vi "ECS-Diesel-Host.vi"() -> ()   [LabVIEW 2015]
uses:
  <vilib>/addons/Software Calibration Management/XControls/SubHost.xctl
  <vilib>/addons/Software Calibration Management/XControls/SubHost List.xctl
  Typedefs/EPT/Engine Status.ctl
  SubHosts/Support/Tracking Chart xCTL/TrackingChart.xctl
  <vilib>/addons/Software Calibration Management/XControls/TBL1D.xctl
  <vilib>/addons/Software Calibration Management/XControls/Faults.xctl
  ECS-Host.lvlib
  ECS-Shared.lvlib
panel:
  out "CalPointData":sgl[](array[numeric])
  in  "_Refresh":bool
  in  "EngineSpeed_MaxNC":sgl
  in  "EngineSpeed_MaxCrit":sgl
  out "5VPSU_CriticalFault":bool
  out "12VPSU_CriticalFault":bool
  out "BattV_CriticalFault":bool
  in  "_Main Tabs":T1(tab)
  in  "PowerEnable":bool caption="Power Enable"
  out "EngineSpeedFPGA1":sgl(knob) scale=0.0..1000.0 scale format="%#_6p"
  in  "SyncEnable":bool caption="Sync Enable"
  out "ReceivingPrimaryFPGA1":bool caption="Rcvg Primary"
  out "SyncFPGA1":bool caption="Sync"
  out "_BattVPresent":bool caption="Battery"
  out "_12VPresent":bool caption="12V"
  out "_5VPresent":bool caption="5V"
  out "Engine Time":sgl caption="[hr]" format="%0#5_4f"
  out "Time Since Start":sgl caption="[sec]" format="%05.0f"
  in  "Engine Time Reset":bool
  out "_Engine Speed":sgl format="%#.0f"
  out "Software Version":string caption="Version:"
  out "_Engine Status":T2 caption="Engine Status"
  in  "Faults Table":T4(xcontrol)
  in  "_SubHost Tab":T5(tab)
  in  "XNET CAN":T6(xcontrol)
  in  "Power":T6(xcontrol)
  in  "TDK High Voltage Supply":T6(xcontrol)
  in  "NI 9754-1 (ESTTL)":T6(xcontrol)
  in  "NI 9411-1 (Digital Input)":T6(xcontrol)
  in  "NI 9758-2 (PFI/LS)":T6(xcontrol)
  in  "NI 9751-4 (DI Driver)":T6(xcontrol)
  in  "NI 9751-3 (DI Driver)":T6(xcontrol)
  in  "NI 9751-2 (DI Driver)":T6(xcontrol)
  in  "NI 9752-1 (ADCombo)":T6(xcontrol)
  in  "NI 9757-1 (O2)":T6(xcontrol)
  in  "NI 9755-1 (NOx)":T6(xcontrol)
  in  "NI 9759-1 (Throttle)":T6(xcontrol)
  in  "NI 9758-1 (PFI/LS)":T6(xcontrol)
  in  "NI 9751-1 (DI Driver)":T6(xcontrol)
  in  "EPTx":T6(xcontrol)
  in  "Sensors":T6(xcontrol)
  in  "Faults":T6(xcontrol) caption="0"
  in  "Engine Specs":T6(xcontrol)
  in  "High Pressure Common Rail":T6(xcontrol)
  in  "Variable Valve Actuation":T6(xcontrol)
  in  "Boost Actuation":T6(xcontrol)
  in  "Direct Injectors":T6(xcontrol)
  in  "EGR Actuation":T6(xcontrol)
  in  "EGR Control":T6(xcontrol) caption="5"
  in  "Cranking":T6(xcontrol) caption="0"
  in  "Wastegate Control":T6(xcontrol) caption="6"
  in  "VGT Control":T6(xcontrol) caption="6"
  in  "Intake Air Desired MAP":T6(xcontrol) caption="5"
  in  "DI Control":T6(xcontrol) caption="2"
  in  "Fuel Command":T6(xcontrol) caption="1"
  in  "Load Command":T6(xcontrol) caption="0"
  in  "Intake Air Measured":T6(xcontrol) caption="1"
  in  "EGR Flow":T6(xcontrol) caption="5"
  in  "VVT/VVA Control":T6(xcontrol) caption="9"
  in  "Rail Pressure Control":T6(xcontrol) caption="4"
  in  "Execution Info":T6(xcontrol)
  in  "Calscope and Trends":T6(xcontrol)
  in  "_HiddenControls":enum32{"Page 1"}(tab)
  out "RailP_Des":sgl
  out "MAP_Des":sgl
  in  "NominalMEP_Tbl":cluster{"X":sgl[], "Y":sgl[]}(xcontrol)
  out "MEP_Des":sgl caption="EngineLoad_Des"
  out "Pedal_Des":sgl
  out "EngineStatus":u8
  in  "_HiddenControls2":enum32{"Page 1"}(tab)
  in  "SliderMin":sgl[](array[numeric])
  in  "SliderMax":sgl[](array[numeric])
  in  "Units":string
  in  "_Signal Names":string[](array[string])
  in  "CalPointIDs":sgl[](array[numeric])
  out "NamesLong":string
  in  "SliderSelection":sgl[](array[numeric])
  in  "MAP_ManE":bool
  in  "Pedal_ManE":bool
  in  "MEP_ManE":bool
  in  "RailP_ManE":bool
  in  "Pedal_Man":sgl(slide) caption="[bar]" scale=0.0..100.0 scale format="%#4.1f"
  in  "MEP_Man":sgl(slide) caption="[bar]" scale=0.0..25.0 scale format="%#4.1f"
  in  "RailP_Man":sgl(slide) caption="[bar]" scale=0.0..2000.0 scale format="%#4.1f"
  in  "MAP_Man":sgl(slide) caption="[kPa]" scale=0.0..400.0 scale format="%#4.1f"
  in  "ForceSafeState":bool caption="Push to Force Safe State"
  out "Non-Critical Fault":bool
  out "Critical Fault":bool
  in  "ESTOP":bool caption="Push to Stop"
  in  "System":T7(xcontrol)
  in  "Control":T7(xcontrol)
  in  "Engine":T7(xcontrol)
  in  "Hardware":T7(xcontrol)
  out "_TrackingChart":T8(xcontrol)
  in  "_Delete":bool
  in  "_Down":bool
  in  "_Up":bool
  in  "_Insert":bool
  out "_Data (Hidden)":string[](array[string])
  in  "_Units":string caption="Units"
  in  "_Slider Max":sgl caption="Max"
  in  "_Slider Min":sgl caption="Min"
  in  "_CalpointIDSelect":u16(ring) caption="Signal Name"
  in  "_Slider Selection":T9(ring) caption="Slider Selection"
  in  "_Table":i32(listbox)
  in  "_Chart History1":i32=20 caption="Chart History"
  out "_LoadTracking":cluster{"X Buffer":sgl[], "Y Buffer":sgl[]}[](graph) caption="Load Tracking"
  in  "_Chart History2":i32=20 caption="Chart History"
  in  "_Normalize":bool=TRUE caption="Normalize"
  in  "_Var Select":u16(ring) caption="Signal Selection" items=["EngineLoad_Des", "InjDur", "InjTiming", "RailP", "RailP_Des", "MAP", "MAP_Des", "MAF", "Lambda", "FuelT", "ECT", "MAT", "OilP", "ExhaustManifoldT", "MainSpkDwell", "MainSpkTiming"]
  out "_ReturnMap":cluster{"X Buffer":sgl[], "Y Buffer":sgl[]}[](graph) caption="Return Map"
  # "Engine Control System"
  # "RPM"
  # "Customize UI Here"
  # "Customize UI Here"
  # "Customize UI Here"
  # "Un-hide from the block diagram by right-clicking '_HiddenControls' and selecting 'Show Control'"
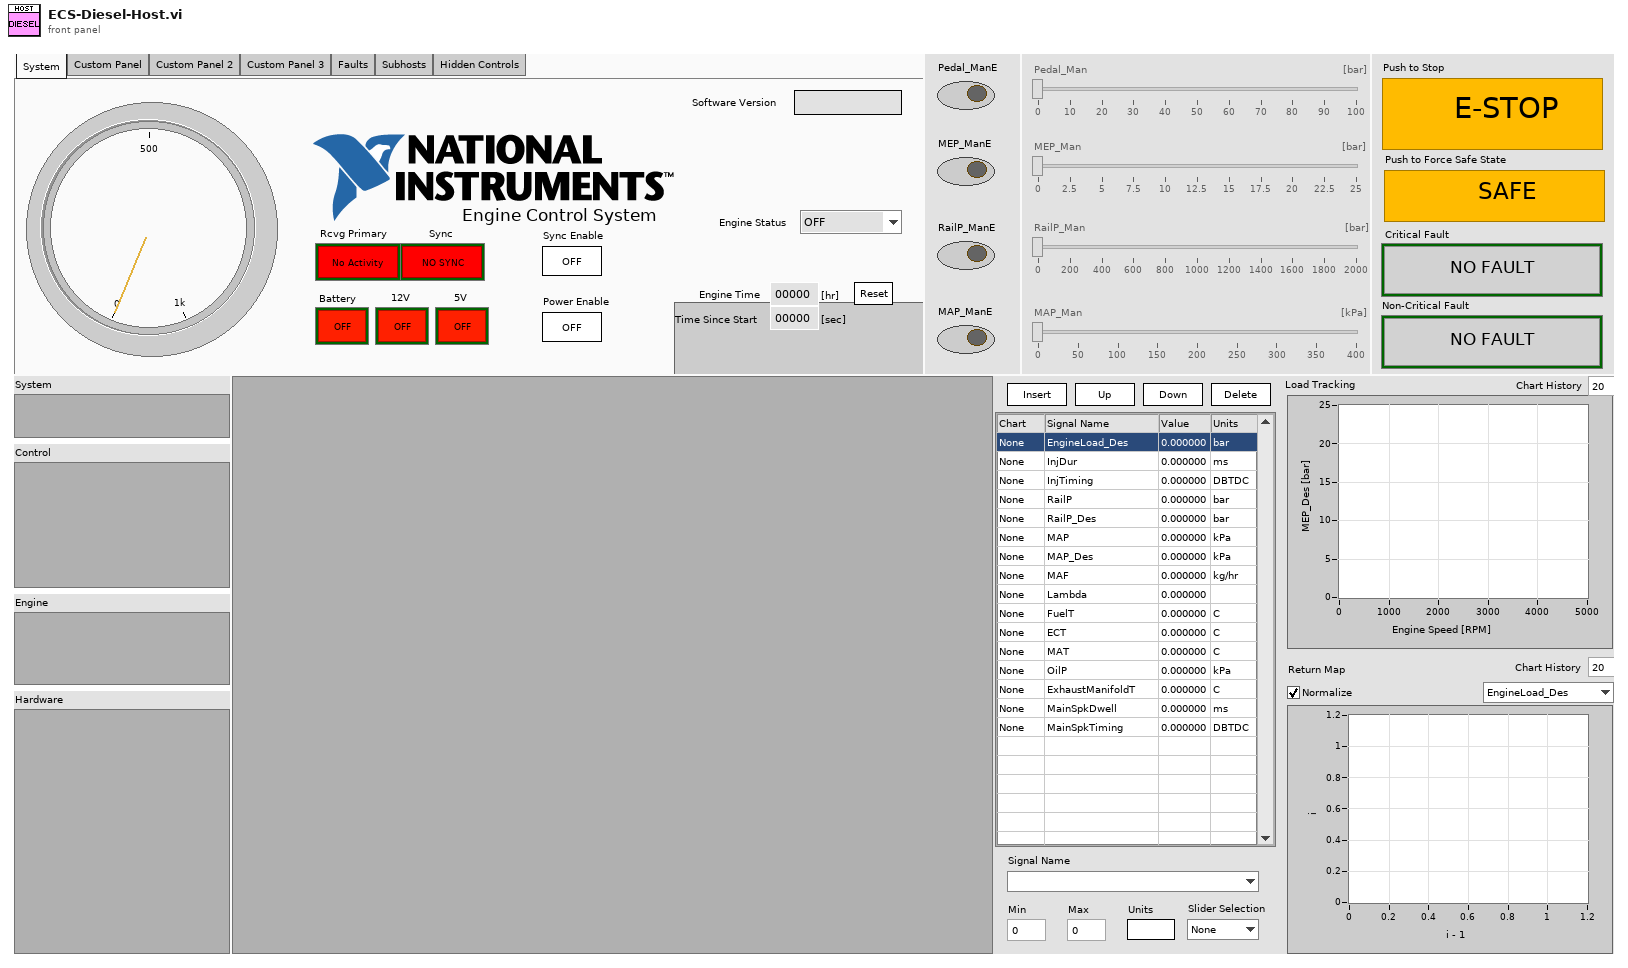
[diagram p1: front panel]
types:
  T1 = enum32{"System", "Custom Panel", "Custom Panel 2", "Custom Panel 3", "Faults", "Subhosts", "Hidden Controls"}
  T2 = typedef "ECS-Shared.lvlib/Engine Status.ctl" = enum16{"OFF", "STALLED", "CRANKING", "RUNNING", "ACCEL", "DECEL", "SAFE"}
  T3 = typedef "Faults.xctl/Faults - Active.ctl" = cluster{"Highest Level":i32, "Very Low":u32, "Low":u32, "Medium":u32, "High":u32, "Very High":u32}
  T4 = cluster{"Active Faults":T3, "Unacknowledged Faults":T3}
  T5 = enum32{"Hardware I/O", "Engine I/O", "Control", "System"}
  T6 = cluster{"Name":string, "Host VI":path, "Pairing File":path, "Display Name":string}
  T7 = cluster{"States":enum32{"Invalid", "Standard", "Closed", "Hidden", "Minimized", "Maximized"}[], "VI Names":string[], "VI Refnums":refnum<vi>[], "Sub-Host Group":string, "Scrollbar":bool, "Listbox":refnum<vi>}
  T8 = cluster{"Value":sgl, "Name":string, "Unit":string, "Max":sgl, "Min":sgl}[]
  T9 = enum16{"None", "Slider 1", "Slider 2", "Slider 3", "Slider 4"}
  T10 = enum8{"Enabled", "Disabled", "Disabled and Grayed Out"}
  T11 = cluster{"Value":sgl, "Name":string, "Unit":string, "Max":sgl, "Min":sgl}
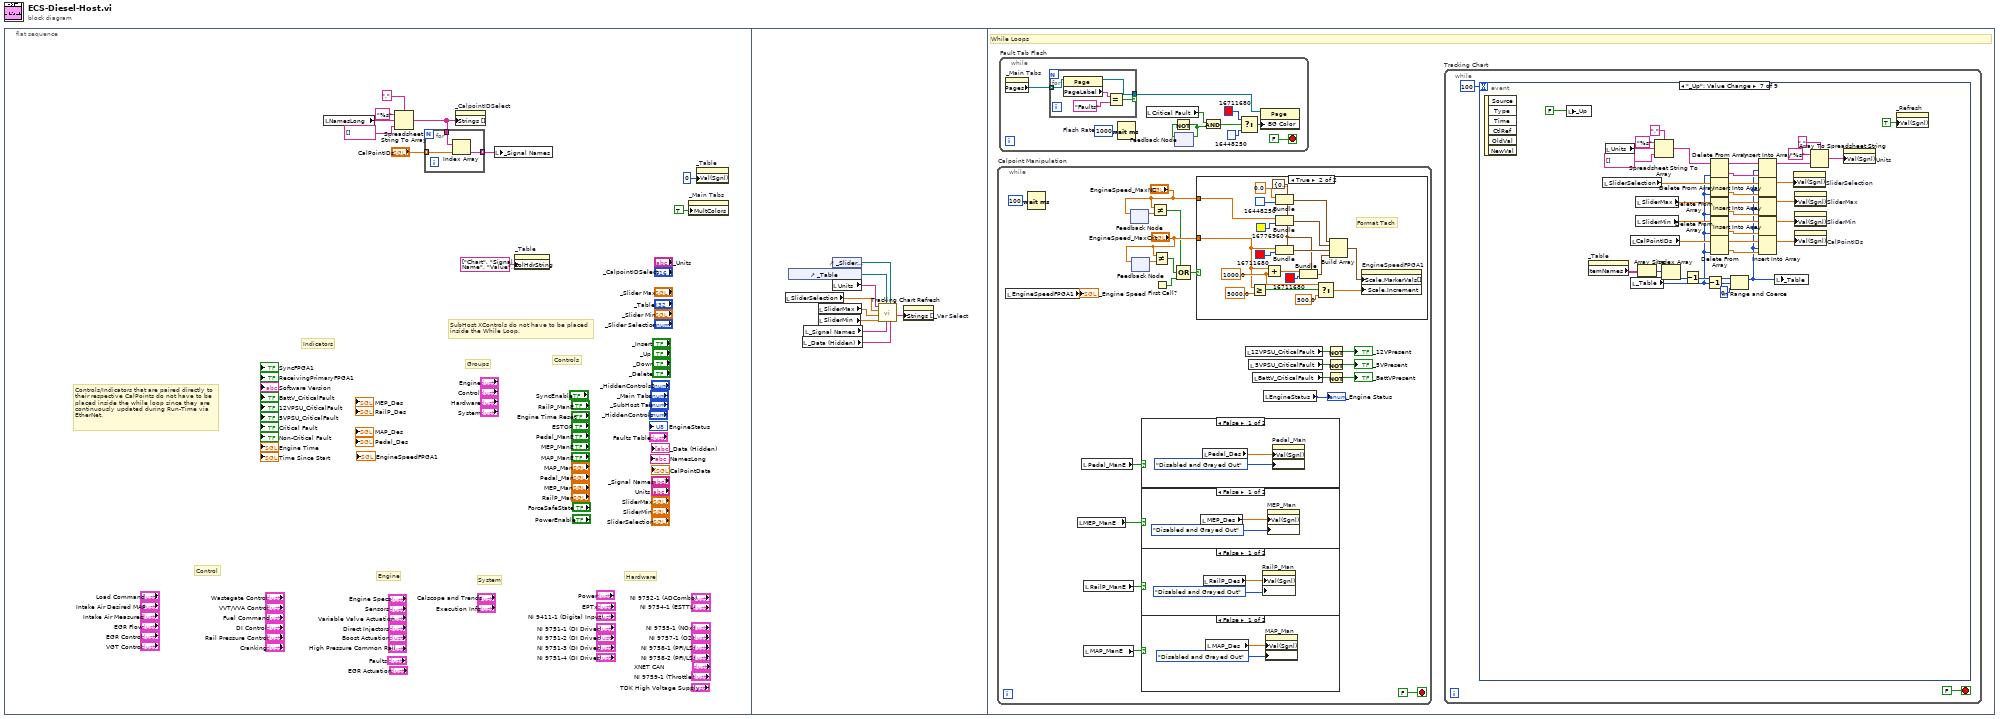
[diagram p0: block diagram]
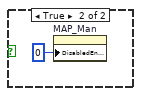
[diagram p2: hidden frame]
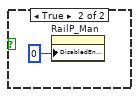
[diagram p3: hidden frame]
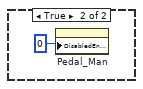
[diagram p4: hidden frame]
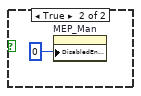
[diagram p5: hidden frame]
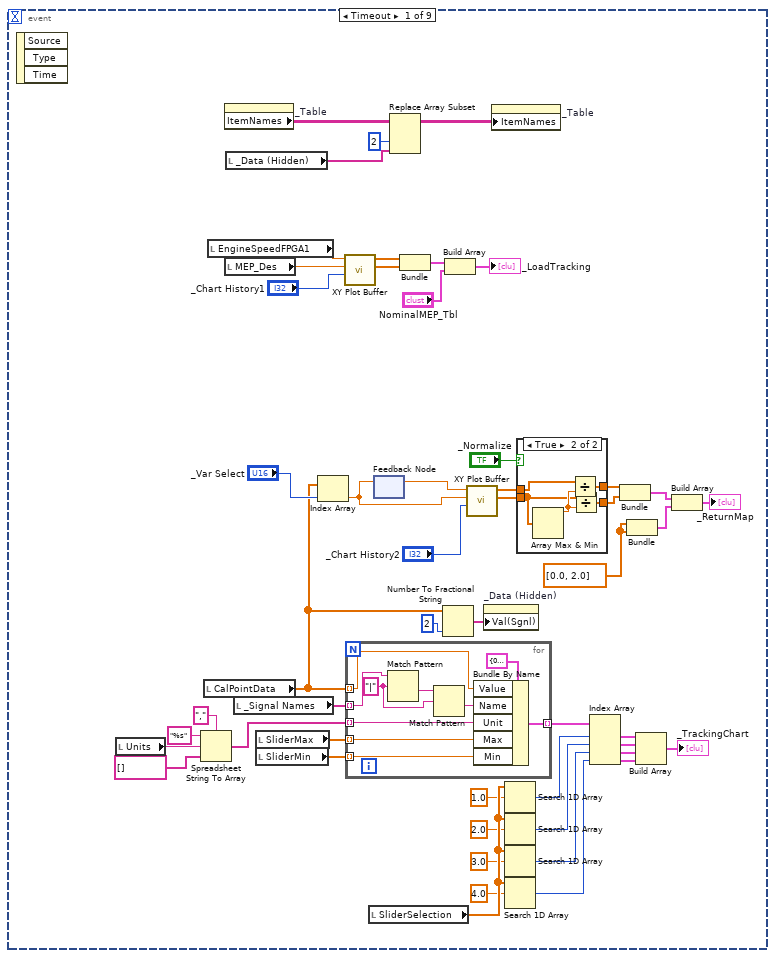
[diagram p7: hidden frame]
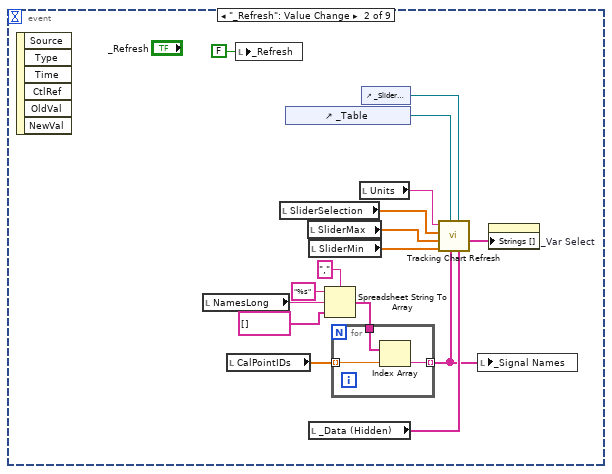
[diagram p9: hidden frame]
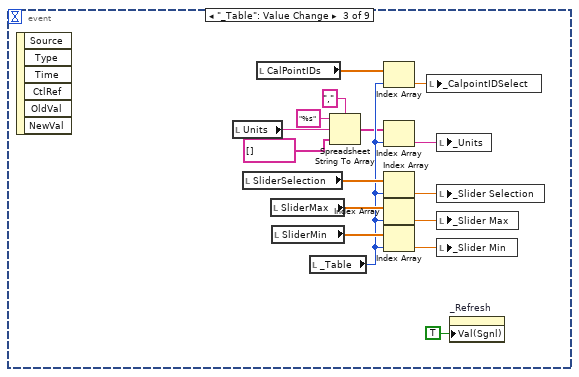
[diagram p10: hidden frame]
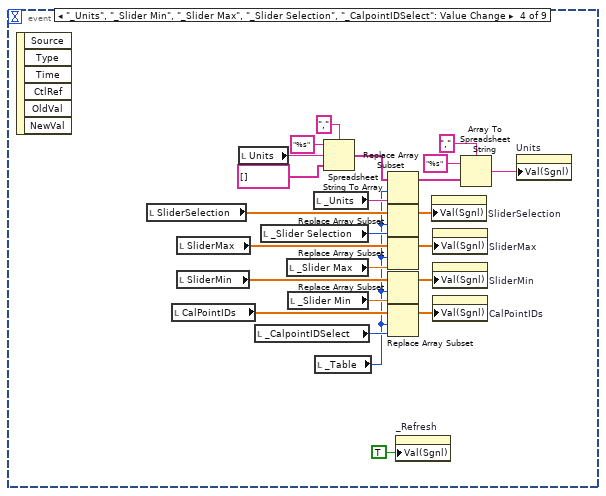
[diagram p11: hidden frame]
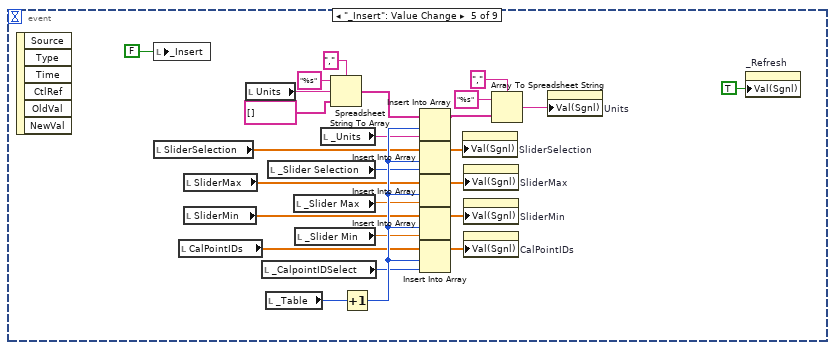
[diagram p12: hidden frame]
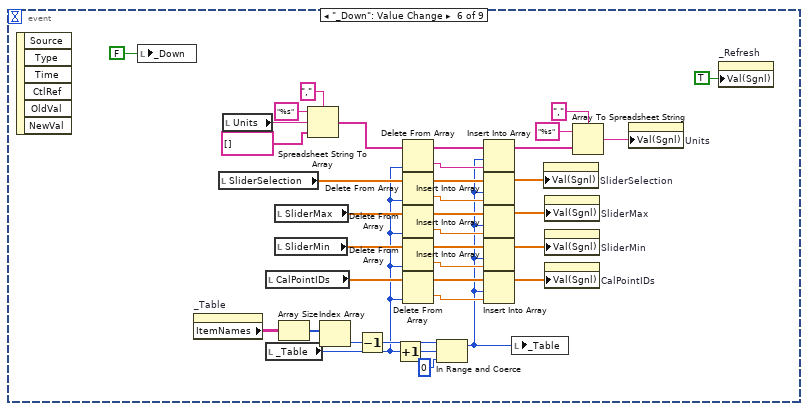
[diagram p13: hidden frame]
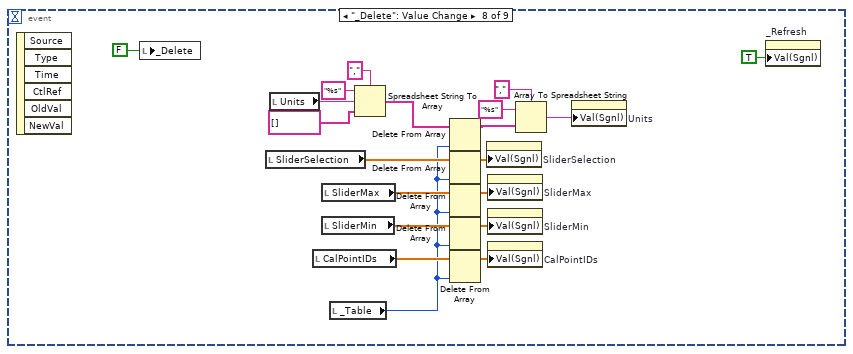
[diagram p14: hidden frame]
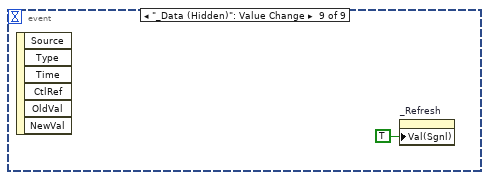
[diagram p15: hidden frame]
diagram:
  n1 = flat-sequence {
    frame #0 {
      # "System"
      # "Hardware"
      # "Engine"
      # "Control"
      # "Controls"
      # "Indicators"
      # "Groups"
      # "Controls/Indicators that are paired directly to their respective CalPoints do not have to be placed inside the while loop since they are continuously updated during Run-Time via EtherNet."
      # "SubHost XControls do not have to be placed inside the While Loop."
      n2 = local read "NamesLong"() -> (w4:string)
      n3 = Spreadsheet String To Array(delimiter (Tab)=",", format string="%s", spreadsheet string=w4, array type (2D Dbl)=string[] []) -> (array=w1:string[])
      n4 = for {
        tunnel: "CalPointIDs" -> [w13] mode=indexing
        tunnel: w1 -> [w12]
        tunnel: [w11] -> w2 mode=indexing
        n5 = Index Array(array=w12, index=w13) -> (element=w11:string)
      }
      n6 = property on="_CalpointIDSelect" class="Ring (strict)"("Strings []"=w1) -> ()  [unwired: 2 in, 2 out]
      n7 = local write "_Signal Names"(w2) -> ()
      n8 = property on="_Table" class="MCListbox (strict)"("ColHdrString"=string[] ["Chart", "Signal Name", "Value", "Units"] ("Column Header Strings[]")) -> ()  [unwired: 2 in, 2 out]
      n9 = property on="_Main Tabs" class="TabCtl (strict)"("MultColors"=TRUE ("Allow Multiple Colors")) -> ()  [unwired: 2 in, 2 out]
      n10 = property on="_Table" class="MCListbox (strict)"("Val(Sgnl)"=0 ("Value (Signaling)")) -> ()  [unwired: 2 in, 2 out]
    }
    frame #1 {
      n11 = local read "SliderSelection"() -> (w20:sgl[])
      n12 = control-ref of="_Table"() -> (w21:refnum<vi>)
      n13 = local read "_Data (Hidden)"() -> (w17:string[])
      n14 = local read "_Signal Names"() -> (w16:string[])
      n15 = local read "SliderMax"() -> (w19:sgl[])
      n16 = local read "SliderMin"() -> (w18:sgl[])
      n17 = local read "Units"() -> (w15:string)
      n18 = control-ref of="_Slider Selection"() -> (w22:refnum<vi>)
      n19 = call "Tracking Chart Refresh.vi"("Data"=w17, "_Slider Selection"=w22, "Signal Names"=w16, "_Table"=w21, "Slider Min"=w18, "Slider Max"=w19, "Slider Selections"=w20, "Units"=w15) -> ("Short Signal Names"=w14:string[])  [unwired: 3 in]
      n20 = property on="_Var Select" class="Ring (strict)"("Strings []"=w14) -> ()  [unwired: 2 in, 2 out]
    }
    frame #2 {
      # "While Loops"
      n21 = while "Calpoint Manipulation" {
        stop <- FALSE stop-if-true
        n22 = local read "EngineSpeedFPGA1"() -> (→"_Engine Speed":sgl)
        n23 = Wait (ms)(milliseconds to wait=u32 100) -> ()  [unwired: 1 out]
        n24 = local read "MEP_ManE"() -> (w43:bool)
        n25 = local read "Pedal_ManE"() -> (w42:bool)
        n26 = local read "RailP_ManE"() -> (w41:bool)
        n27 = local read "MAP_ManE"() -> (w40:bool)
        n28 = feedback #1() -> (w49:sgl)  [unwired: 1 in]
        n29 = feedback-in #1("EngineSpeed_MaxNC") -> ()
        n30 = feedback #2() -> (w57:sgl)  [unwired: 1 in]
        n31 = feedback-in #2("EngineSpeed_MaxCrit") -> ()
        n32 = case shown="False" w42 {
          frame False {
            n33 = local read "Pedal_Des"() -> (w67:sgl)
            n34 = property on="Pedal_Man" class="Slide (strict)"("Val(Sgnl)"=w67, "DisabledEnum"=T10."Disabled and Grayed Out" ("Disabled")) -> ()  [unwired: 2 in, 2 out]
          }
          frame True {
            n35 = property on="Pedal_Man" class="Slide (strict)"("DisabledEnum"=u8 0) -> ()  [unwired: 2 in, 2 out]
          }
        }
        n36 = case shown="False" w43 {
          frame False {
            n37 = local read "MEP_Des"() -> (w71:sgl)
            n38 = property on="MEP_Man" class="Slide (strict)"("Val(Sgnl)"=w71, "DisabledEnum"=T10."Disabled and Grayed Out" ("Disabled")) -> ()  [unwired: 2 in, 2 out]
          }
          frame True {
            n39 = property on="MEP_Man" class="Slide (strict)"("DisabledEnum"=u8 0) -> ()  [unwired: 2 in, 2 out]
          }
        }
        n40 = case shown="False" w41 {
          frame False {
            n41 = local read "RailP_Des"() -> (w64:sgl)
            n42 = property on="RailP_Man" class="Slide (strict)"("Val(Sgnl)"=w64, "DisabledEnum"=T10."Disabled and Grayed Out" ("Disabled")) -> ()  [unwired: 2 in, 2 out]
          }
          frame True {
            n43 = property on="RailP_Man" class="Slide (strict)"("DisabledEnum"=u8 0) -> ()  [unwired: 2 in, 2 out]
          }
        }
        n44 = case shown="False" w40 {
          frame False {
            n45 = local read "MAP_Des"() -> (w61:sgl)
            n46 = property on="MAP_Man" class="Slide (strict)"("Val(Sgnl)"=w61, "DisabledEnum"=T10."Disabled and Grayed Out" ("Disabled")) -> ()  [unwired: 2 in, 2 out]
          }
          frame True {
            n47 = property on="MAP_Man" class="Slide (strict)"("DisabledEnum"=u8 0) -> ()  [unwired: 2 in, 2 out]
          }
        }
        n48 = Not Equal?(x="EngineSpeed_MaxNC", y=w49) -> (x != y?=w46:bool)
        n49 = Not Equal?(x="EngineSpeed_MaxCrit", y=w57) -> (x != y?=w45:bool)
        n50 = First Call?() -> (First Call?: T/F=w47:bool)
        n51 = Compound Arithmetic op=OR(w46, w45, w47) -> (w48:bool)
        n52 = case shown="True" w48 {
          tunnel: "EngineSpeed_MaxCrit" -> [_ w80]
          tunnel: "EngineSpeed_MaxNC" -> [_ w74]
          frame False {
          }
          frame True {
            w81 = sgl 1000.0 ("y")
            w77 = cluster{dbl, u32} {0.0, 0}
            # "Format Tach"
            n53 = Greater Or Equal?(x=w80, y=sgl 5000.0) -> (x >= y?=w83:bool)
            n54 = Add(x=w80, y=w81) -> (x+y=w85:sgl)
            n55 = Bundle(cluster=w77, sgl 0.0, u32 16448250) -> (w76:cluster{dbl, u32})
            n56 = Bundle(cluster=w77, w74, u32 16776960) -> (w75:cluster{dbl, u32})
            n57 = Bundle(cluster=w77, w80, u32 16711680) -> (w91:cluster{dbl, u32})
            n58 = Bundle(cluster=w77, w85, u32 16711680) -> (w88:cluster{dbl, u32})
            n59 = Select(t=w81, s=w83, f=sgl 500.0 ("Scale.Range:Increment")) -> (s? t:f=w78:sgl)
            n60 = Build Array(w76, w75, w91, w88) -> (w79:cluster{dbl, u32}[])
            n61 = property on="EngineSpeedFPGA1" class="Knob (strict)"("Scale.MarkerVals[]"=w79, "Scale.Increment"=w78) -> ()  [unwired: 2 in, 2 out]
          }
        }
        n62 = local read "12VPSU_CriticalFault"() -> (w53:bool)
        n63 = local read "5VPSU_CriticalFault"() -> (w54:bool)
        n64 = local read "BattV_CriticalFault"() -> (w55:bool)
        n65 = local read "EngineStatus"() -> (→"_Engine Status":u8)
        n66 = Not(x=w53) -> (.not. x?=→"_12VPresent":bool)
        n67 = Not(x=w54) -> (.not. x?=→"_5VPresent":bool)
        n68 = Not(x=w55) -> (.not. x?=→"_BattVPresent":bool)
      }
      n69 = while "Fault Tab Flash" {
        stop <- FALSE stop-if-true
        w32 = u32 1000  # Flash Rate
        n70 = property on="_Main Tabs" class="TabCtl (strict)"() -> ("Pages"=w24:refnum<vi>[])  [unwired: 2 in, 2 out]
        n71 = for {
          tunnel: w24 -> [w38] mode=indexing
          tunnel: [w34] -> w23 if=w35
          n72 = property class="Page"(reference=w38) -> (reference out=w34:refnum<vi>, "PageLabel"=w37:string)  [unwired: 1 in, 1 out]
          n73 = Equal?(x=w37, y="Faults") -> (x = y?=w35:bool)
        }
        n74 = Wait (ms)(milliseconds to wait=w32) -> ()  [unwired: 1 out]
        n75 = local read "Critical Fault"() -> (w25:bool)
        n76 = feedback #3() -> (w29:bool)  [unwired: 1 in]
        n77 = Not(x=w29) -> (.not. x?=w30:bool)
        n78 = feedback-in #3(w30) -> ()
        n79 = And(x=w25, y=w30) -> (x .and. y?=w28:bool)
        n80 = Select(t=u32 16711680, s=w28, f=u32 16448250) -> (s? t:f=w27:u32)
        n81 = property class="Page"(reference=w23, "BG Color"=w27) -> ()  [unwired: 1 in, 2 out]
      }
      n82 = while "Tracking Chart" {
        stop <- FALSE stop-if-true
        n83 = event shown="[6] \"_Up\": Value Change" {
          selector: _ -> [_ _ _ _ _ _ _ _ _]
          dyn-events: _ -> [_ _ _ _ _ _ _ _ _]
          timeout: 100 -> [_ _ _ _ _ _ _ _ _]
          event Timeout {
            w127 = sgl[] [0.0, 2.0]
            n84 = event-data() -> ()  [unwired: 1 in, 3 out]
            n85 = local read "Units"() -> (w101:string)
            n86 = Spreadsheet String To Array(delimiter (Tab)=",", format string="%s", spreadsheet string=w101, array type (2D Dbl)=string[] []) -> (array=w102:string[])
            n87 = local read "CalPointData"() -> (w106:sgl[])
            n88 = local read "EngineSpeedFPGA1"() -> (w134:sgl)
            n89 = property on="_Table" class="MCListbox (strict)"() -> ("ItemNames"=w144:string[][])  [unwired: 2 in, 2 out]
            n90 = local read "MEP_Des"() -> (w133:sgl)
            n91 = local read "_Data (Hidden)"() -> (w143:string[])
            n92 = local read "_Signal Names"() -> (w98:string[])
            n93 = local read "SliderMax"() -> (w100:sgl[])
            n94 = local read "SliderMin"() -> (w99:sgl[])
            n95 = Index Array(array=w106, index="_Var Select") -> (element=w132:sgl)
            n96 = call "XY Plot Buffer.vi"("History Length"="_Chart History1", "Input 2"=w133, "Input 1"=w134) -> ("Y Buffer"=w136:sgl[], "X Buffer"=w137:sgl[])  [unwired: 7 in]
            n97 = for {
              tunnel: w106 -> [w149] mode=indexing
              tunnel: w102 -> [w154] mode=indexing
              tunnel: w100 -> [w153] mode=indexing
              tunnel: w99 -> [w152] mode=indexing
              tunnel: [w151] -> w115 mode=indexing
              tunnel: w98 -> [w145] mode=indexing
              w147 = "|" ("regular expression")
              n98 = Match Pattern(string=w145, regular expression=w147) -> (after substring=w148:string)  [unwired: 1 in, 3 out]
              n99 = Match Pattern(string=w148, regular expression=w147) -> (after substring=w146:string)  [unwired: 1 in, 3 out]
              n100 = Bundle By Name(cluster=T11 {"Value"=0.0, "Name"="", "Unit"="", "Max"=0.0, "Min"=0.0} ("Data"), "Value"=w149, "Name"=w146, "Unit"=w154, "Max"=w153, "Min"=w152) -> (w151:T11)
            }
            n101 = local read "SliderSelection"() -> (w114:sgl[])
            n102 = feedback #4() -> (w131:sgl)  [unwired: 1 in]
            n103 = feedback-in #4(w132) -> ()
            n104 = Replace Array Subset(array=w144, new element=w143, index (col)=2 ("disabled index (col)")) -> (w141:string[][])  [unwired: 1 in]
            n105 = Bundle("X Buffer"=w137, "Y Buffer"=w136) -> (w139:cluster{"X Buffer":sgl[], "Y Buffer":sgl[]})  [unwired: 1 in]
            n106 = Number To Fractional String(number=w106, precision (6)=i16 2) -> (F-format string=w108:string[])  [unwired: 2 in]
            n107 = Build Array(w139, "NominalMEP_Tbl") -> (→"_LoadTracking":cluster{"X":sgl[], "Y":sgl[]}[])
            n108 = call "XY Plot Buffer.vi"("History Length"="_Chart History2", "Input 2"=w132, "Input 1"=w131) -> ("Y Buffer"=w112:sgl[], "X Buffer"=w110:sgl[])  [unwired: 7 in]
            n109 = property on="_Data (Hidden)" class="Arr (strict)"("Val(Sgnl)"=w108) -> ()  [unwired: 2 in, 2 out]
            n110 = property on="_Table" class="MCListbox (strict)"("ItemNames"=w141) -> ()  [unwired: 2 in, 2 out]
            n111 = Search 1D Array(1D array=w114, element=sgl 1.0) -> (index of element=w116:i32)  [unwired: 1 in]
            n112 = Search 1D Array(1D array=w114, element=sgl 2.0) -> (index of element=w117:i32)  [unwired: 1 in]
            n113 = Search 1D Array(1D array=w114, element=sgl 3.0) -> (index of element=w118:i32)  [unwired: 1 in]
            n114 = Search 1D Array(1D array=w114, element=sgl 4.0) -> (index of element=w119:i32)  [unwired: 1 in]
            n115 = case shown="True" "_Normalize" {
              tunnel: [w156 w161] -> w109
              tunnel: w110 -> [w156 w160]
              tunnel: [w155 w158] -> w111
              tunnel: w112 -> [w155 w157]
              frame False {
              }
              frame True {
                n116 = Array Max & Min(array=w157) -> (max value=w159:sgl)  [unwired: 3 out]
                n117 = Divide(x=w160, y=w159) -> (x/y=w161:sgl[])
                n118 = Divide(x=w157, y=w159) -> (x/y=w158:sgl[])
              }
            }
            n119 = Index Array(array=w115, index #1=w116, index #2=w117, index #3=w118, index #4=w119) -> (element #1=w120:T11, element #2=w121:T11, element #3=w122:T11, element #4=w123:T11)
            n120 = Bundle("X Buffer"=w109, "Y Buffer"=w111) -> (w128:cluster{"X Buffer":sgl[], "Y Buffer":sgl[]})  [unwired: 1 in]
            n121 = Bundle(w127, w127) -> (w129:cluster{sgl[], sgl[]})  [unwired: 1 in]
            n122 = Build Array(w120, w121, w122, w123) -> (→"_TrackingChart":T8)
            n123 = Build Array(w128, w129) -> (→"_ReturnMap":cluster{"X Buffer":sgl[], "Y Buffer":sgl[]}[])
          }
          event "_Refresh": Value Change {
            n124 = event-data() -> ()  [unwired: 1 in, 6 out]
            n125 = local read "NamesLong"() -> (w167:string)
            n126 = local read "CalPointIDs"() -> (w165:sgl[])
            n127 = local write "_Refresh"(FALSE ("_Refresh")) -> ()
            n128 = local read "SliderSelection"() -> (w174:sgl[])
            n129 = control-ref of="_Table"() -> (w175:refnum<vi>)
            n130 = local read "SliderMax"() -> (w173:sgl[])
            n131 = local read "SliderMin"() -> (w172:sgl[])
            n132 = local read "_Data (Hidden)"() -> (w171:string[])
            n133 = Spreadsheet String To Array(delimiter (Tab)=",", format string="%s", spreadsheet string=w167, array type (2D Dbl)=string[] []) -> (array=w166:string[])
            n134 = for {
              tunnel: w165 -> [w180] mode=indexing
              tunnel: w166 -> [w179]
              tunnel: [w178] -> w163 mode=indexing
              n135 = Index Array(array=w179, index=w180) -> (element=w178:string)
            }
            n136 = local read "Units"() -> (w164:string)
            n137 = control-ref of="_Slider Selection"() -> (w176:refnum<vi>)
            n138 = call "Tracking Chart Refresh.vi"("Data"=w171, "_Slider Selection"=w176, "Signal Names"=w163, "_Table"=w175, "Slider Min"=w172, "Slider Max"=w173, "Slider Selections"=w174, "Units"=w164) -> ("Short Signal Names"=w162:string[])  [unwired: 3 in]
            n139 = local write "_Signal Names"(w163) -> ()
            n140 = property on="_Var Select" class="Ring (strict)"("Strings []"=w162) -> ()  [unwired: 2 in, 2 out]
          }
          event "_Table": Value Change {
            n141 = event-data() -> ()  [unwired: 1 in, 6 out]
            n142 = local read "Units"() -> (w182:string)
            n143 = local read "SliderSelection"() -> (w196:sgl[])
            n144 = local read "CalPointIDs"() -> (w189:sgl[])
            n145 = local read "SliderMax"() -> (w195:sgl[])
            n146 = local read "SliderMin"() -> (w194:sgl[])
            n147 = local read "_Table"() -> (w187:i32)
            n148 = Spreadsheet String To Array(delimiter (Tab)=",", format string="%s", spreadsheet string=w182, array type (2D Dbl)=string[] []) -> (array=w183:string[])
            n149 = Index Array(array=w189, index=w187) -> (element=w181:sgl)
            n150 = Index Array(array=w183, index=w187) -> (element=w193:string)
            n151 = Index Array(array=w196, index=w187) -> (element=w192:sgl)
            n152 = Index Array(array=w195, index=w187) -> (element=w191:sgl)
            n153 = Index Array(array=w194, index=w187) -> (element=w190:sgl)
            n154 = local write "_CalpointIDSelect"(w181) -> ()
            n155 = local write "_Units"(w193) -> ()
            n156 = local write "_Slider Selection"(w192) -> ()
            n157 = local write "_Slider Max"(w191) -> ()
            n158 = local write "_Slider Min"(w190) -> ()
            n159 = property on="_Refresh" class="Bool (strict)"("Val(Sgnl)"=TRUE ("Value (Signaling)")) -> ()  [unwired: 2 in, 2 out]
          }
          event "_Units", "_Slider Min", "_Slider Max", "_Slider Selection", "_CalpointIDSelect": Value Change {
            n160 = event-data() -> ()  [unwired: 1 in, 6 out]
            n161 = local read "SliderSelection"() -> (w216:sgl[])
            n162 = local read "CalPointIDs"() -> (w198:sgl[])
            n163 = local read "SliderMax"() -> (w217:sgl[])
            n164 = local read "SliderMin"() -> (w220:sgl[])
            n165 = local read "Units"() -> (w206:string)
            n166 = local read "_CalpointIDSelect"() -> (w199:u16)
            n167 = local read "_Slider Selection"() -> (w215:T9)
            n168 = local read "_Slider Max"() -> (w218:sgl)
            n169 = local read "_Slider Min"() -> (w219:sgl)
            n170 = local read "_Units"() -> (w214:string)
            n171 = local read "_Table"() -> (w197:i32)
            n172 = Spreadsheet String To Array(delimiter (Tab)=",", format string="%s", spreadsheet string=w206, array type (2D Dbl)=string[] []) -> (array=w205:string[])
            n173 = Replace Array Subset(array=w205, new element=w214, index=w197) -> (w202:string[])
            n174 = Replace Array Subset(array=w216, new element=w215, index=w197) -> (w211:sgl[])
            n175 = Replace Array Subset(array=w217, new element=w218, index=w197) -> (w213:sgl[])
            n176 = Replace Array Subset(array=w220, new element=w219, index=w197) -> (w212:sgl[])
            n177 = Replace Array Subset(array=w198, new element=w199, index=w197) -> (w200:sgl[])
            n178 = property on="_Refresh" class="Bool (strict)"("Val(Sgnl)"=TRUE ("Value (Signaling)")) -> ()  [unwired: 2 in, 2 out]
            n179 = property on="SliderSelection" class="Arr (strict)"("Val(Sgnl)"=w211) -> ()  [unwired: 2 in, 2 out]
            n180 = property on="SliderMax" class="Arr (strict)"("Val(Sgnl)"=w213) -> ()  [unwired: 2 in, 2 out]
            n181 = property on="SliderMin" class="Arr (strict)"("Val(Sgnl)"=w212) -> ()  [unwired: 2 in, 2 out]
            n182 = property on="CalPointIDs" class="Arr (strict)"("Val(Sgnl)"=w200) -> ()  [unwired: 2 in, 2 out]
            n183 = Array To Spreadsheet String(delimiter (Tab)=",", array=w202, 3:"%s" ("format string")) -> (spreadsheet string=w201:string)
            n184 = property on="Units" class="Str"("Val(Sgnl)"=w201) -> ()  [unwired: 2 in, 2 out]
          }
          event "_Insert": Value Change {
            n185 = event-data() -> ()  [unwired: 1 in, 6 out]
            n186 = local write "_Insert"(FALSE ("_Refresh")) -> ()
            n187 = local read "SliderSelection"() -> (w228:sgl[])
            n188 = local read "CalPointIDs"() -> (w225:sgl[])
            n189 = local read "SliderMax"() -> (w227:sgl[])
            n190 = local read "SliderMin"() -> (w226:sgl[])
            n191 = local read "Units"() -> (w242:string)
            n192 = local read "_CalpointIDSelect"() -> (w224:u16)
            n193 = local read "_Table"() -> (w233:i32)
            n194 = local read "_Slider Selection"() -> (w229:T9)
            n195 = local read "_Slider Max"() -> (w231:sgl)
            n196 = local read "_Slider Min"() -> (w230:sgl)
            n197 = local read "_Units"() -> (w222:string)
            n198 = Spreadsheet String To Array(delimiter (Tab)=",", format string="%s", spreadsheet string=w242, array type (2D Dbl)=string[] []) -> (array=w223:string[])
            n199 = Increment(x=w233) -> (x+1=w232:i32)
            n200 = Insert Into Array(array=w223, index=w232, new element=w222) -> (w234:string[])
            n201 = Insert Into Array(array=w228, index=w232, new element=w229) -> (w235:sgl[])
            n202 = Insert Into Array(array=w227, index=w232, new element=w231) -> (w236:sgl[])
            n203 = Insert Into Array(array=w226, index=w232, new element=w230) -> (w237:sgl[])
            n204 = Insert Into Array(array=w225, index=w232, new element=w224) -> (w238:sgl[])
            n205 = property on="SliderSelection" class="Arr (strict)"("Val(Sgnl)"=w235) -> ()  [unwired: 2 in, 2 out]
            n206 = property on="SliderMax" class="Arr (strict)"("Val(Sgnl)"=w236) -> ()  [unwired: 2 in, 2 out]
            n207 = property on="SliderMin" class="Arr (strict)"("Val(Sgnl)"=w237) -> ()  [unwired: 2 in, 2 out]
            n208 = property on="CalPointIDs" class="Arr (strict)"("Val(Sgnl)"=w238) -> ()  [unwired: 2 in, 2 out]
            n209 = Array To Spreadsheet String(delimiter (Tab)=",", array=w234, 3:"%s" ("format string")) -> (spreadsheet string=w239:string)
            n210 = property on="Units" class="Str"("Val(Sgnl)"=w239) -> ()  [unwired: 2 in, 2 out]
            n211 = property on="_Refresh" class="Bool (strict)"("Val(Sgnl)"=TRUE ("Value (Signaling)")) -> ()  [unwired: 2 in, 2 out]
          }
          event "_Down": Value Change {
            n212 = event-data() -> ()  [unwired: 1 in, 6 out]
            n213 = local write "_Down"(FALSE ("_Refresh")) -> ()
            n214 = property on="_Table" class="MCListbox (strict)"() -> ("ItemNames"=w250:string[][])  [unwired: 2 in, 2 out]
            n215 = local read "SliderSelection"() -> (w273:sgl[])
            n216 = local read "Units"() -> (w280:string)
            n217 = local read "CalPointIDs"() -> (w275:sgl[])
            n218 = local read "_Table"() -> (w264:i32)
            n219 = local read "SliderMax"() -> (w272:sgl[])
            n220 = local read "SliderMin"() -> (w271:sgl[])
            n221 = Array Size(array=w250) -> (size(s)=w267:i32[])
            n222 = Spreadsheet String To Array(delimiter (Tab)=",", format string="%s", spreadsheet string=w280, array type (2D Dbl)=string[] []) -> (array=w274:string[])
            n223 = Index Array(array=w267) -> (element=w266:i32)  [unwired: 1 in]
            n224 = Decrement(x=w266) -> (x-1=w269:i32)
            n225 = Increment(x=w264) -> (x+1=w268:i32)
            n226 = Delete From Array(array=w274, index=w264) -> (deleted portion=w263:string, array with subset deleted=w265:string[])  [unwired: 1 in]
            n227 = Delete From Array(array=w273, index=w264) -> (deleted portion=w262:sgl, array with subset deleted=w253:sgl[])  [unwired: 1 in]
            n228 = Delete From Array(array=w272, index=w264) -> (deleted portion=w261:sgl, array with subset deleted=w252:sgl[])  [unwired: 1 in]
            n229 = Delete From Array(array=w271, index=w264) -> (deleted portion=w260:sgl, array with subset deleted=w258:sgl[])  [unwired: 1 in]
            n230 = Delete From Array(array=w275, index=w264) -> (deleted portion=w259:sgl, array with subset deleted=w251:sgl[])  [unwired: 1 in]
            n231 = In Range and Coerce(upper limit=w269, x=w268, lower limit=0) -> (coerced(x)=w249:i32)  [unwired: 1 out]
            n232 = Insert Into Array(array=w265, index=w249, new element=w263) -> (w247:string[])
            n233 = Insert Into Array(array=w253, index=w249, new element=w262) -> (w254:sgl[])
            n234 = Insert Into Array(array=w252, index=w249, new element=w261) -> (w255:sgl[])
            n235 = Insert Into Array(array=w258, index=w249, new element=w260) -> (w257:sgl[])
            n236 = Insert Into Array(array=w251, index=w249, new element=w259) -> (w256:sgl[])
            n237 = local write "_Table"(w249) -> ()
            n238 = property on="SliderSelection" class="Arr (strict)"("Val(Sgnl)"=w254) -> ()  [unwired: 2 in, 2 out]
            n239 = property on="SliderMax" class="Arr (strict)"("Val(Sgnl)"=w255) -> ()  [unwired: 2 in, 2 out]
            n240 = property on="SliderMin" class="Arr (strict)"("Val(Sgnl)"=w257) -> ()  [unwired: 2 in, 2 out]
            n241 = property on="CalPointIDs" class="Arr (strict)"("Val(Sgnl)"=w256) -> ()  [unwired: 2 in, 2 out]
            n242 = Array To Spreadsheet String(delimiter (Tab)=",", array=w247, 3:"%s" ("format string")) -> (spreadsheet string=w277:string)
            n243 = property on="Units" class="Str"("Val(Sgnl)"=w277) -> ()  [unwired: 2 in, 2 out]
            n244 = property on="_Refresh" class="Bool (strict)"("Val(Sgnl)"=TRUE ("Value (Signaling)")) -> ()  [unwired: 2 in, 2 out]
          }
          event "_Up": Value Change {
            n245 = event-data() -> ()  [unwired: 1 in, 6 out]
            n246 = local write "_Up"(FALSE ("_Refresh")) -> ()
            n247 = property on="_Table" class="MCListbox (strict)"() -> ("ItemNames"=w287:string[][])  [unwired: 2 in, 2 out]
            n248 = local read "SliderSelection"() -> (w310:sgl[])
            n249 = local read "Units"() -> (w317:string)
            n250 = local read "CalPointIDs"() -> (w312:sgl[])
            n251 = local read "_Table"() -> (w301:i32)
            n252 = local read "SliderMax"() -> (w309:sgl[])
            n253 = local read "SliderMin"() -> (w308:sgl[])
            n254 = Array Size(array=w287) -> (size(s)=w304:i32[])
            n255 = Spreadsheet String To Array(delimiter (Tab)=",", format string="%s", spreadsheet string=w317, array type (2D Dbl)=string[] []) -> (array=w311:string[])
            n256 = Index Array(array=w304) -> (element=w303:i32)  [unwired: 1 in]
            n257 = Decrement(x=w303) -> (x-1=w306:i32)
            n258 = Decrement(x=w301) -> (x-1=w305:i32)
            n259 = Delete From Array(array=w311, index=w301) -> (deleted portion=w300:string, array with subset deleted=w302:string[])  [unwired: 1 in]
            n260 = Delete From Array(array=w310, index=w301) -> (deleted portion=w299:sgl, array with subset deleted=w290:sgl[])  [unwired: 1 in]
            n261 = Delete From Array(array=w309, index=w301) -> (deleted portion=w298:sgl, array with subset deleted=w289:sgl[])  [unwired: 1 in]
            n262 = Delete From Array(array=w308, index=w301) -> (deleted portion=w297:sgl, array with subset deleted=w295:sgl[])  [unwired: 1 in]
            n263 = Delete From Array(array=w312, index=w301) -> (deleted portion=w296:sgl, array with subset deleted=w288:sgl[])  [unwired: 1 in]
            n264 = In Range and Coerce(upper limit=w306, x=w305, lower limit=0) -> (coerced(x)=w286:i32)  [unwired: 1 out]
            n265 = Insert Into Array(array=w302, index=w286, new element=w300) -> (w284:string[])
            n266 = Insert Into Array(array=w290, index=w286, new element=w299) -> (w291:sgl[])
            n267 = Insert Into Array(array=w289, index=w286, new element=w298) -> (w292:sgl[])
            n268 = Insert Into Array(array=w295, index=w286, new element=w297) -> (w294:sgl[])
            n269 = Insert Into Array(array=w288, index=w286, new element=w296) -> (w293:sgl[])
            n270 = local write "_Table"(w286) -> ()
            n271 = property on="SliderSelection" class="Arr (strict)"("Val(Sgnl)"=w291) -> ()  [unwired: 2 in, 2 out]
            n272 = property on="SliderMax" class="Arr (strict)"("Val(Sgnl)"=w292) -> ()  [unwired: 2 in, 2 out]
            n273 = property on="SliderMin" class="Arr (strict)"("Val(Sgnl)"=w294) -> ()  [unwired: 2 in, 2 out]
            n274 = property on="CalPointIDs" class="Arr (strict)"("Val(Sgnl)"=w293) -> ()  [unwired: 2 in, 2 out]
            n275 = Array To Spreadsheet String(delimiter (Tab)=",", array=w284, 3:"%s" ("format string")) -> (spreadsheet string=w314:string)
            n276 = property on="Units" class="Str"("Val(Sgnl)"=w314) -> ()  [unwired: 2 in, 2 out]
            n277 = property on="_Refresh" class="Bool (strict)"("Val(Sgnl)"=TRUE ("Value (Signaling)")) -> ()  [unwired: 2 in, 2 out]
          }
          event "_Delete": Value Change {
            n278 = event-data() -> ()  [unwired: 1 in, 6 out]
            n279 = local write "_Delete"(FALSE ("_Refresh")) -> ()
            n280 = local read "SliderSelection"() -> (w325:sgl[])
            n281 = local read "Units"() -> (w337:string)
            n282 = local read "CalPointIDs"() -> (w332:sgl[])
            n283 = local read "SliderMax"() -> (w324:sgl[])
            n284 = local read "SliderMin"() -> (w323:sgl[])
            n285 = local read "_Table"() -> (w322:i32)
            n286 = Spreadsheet String To Array(delimiter (Tab)=",", format string="%s", spreadsheet string=w337, array type (2D Dbl)=string[] []) -> (array=w326:string[])
            n287 = Delete From Array(array=w326, index=w322) -> (array with subset deleted=w331:string[])  [unwired: 1 in, 1 out]
            n288 = Delete From Array(array=w325, index=w322) -> (array with subset deleted=w330:sgl[])  [unwired: 1 in, 1 out]
            n289 = Delete From Array(array=w324, index=w322) -> (array with subset deleted=w329:sgl[])  [unwired: 1 in, 1 out]
            n290 = Delete From Array(array=w323, index=w322) -> (array with subset deleted=w328:sgl[])  [unwired: 1 in, 1 out]
            n291 = Delete From Array(array=w332, index=w322) -> (array with subset deleted=w327:sgl[])  [unwired: 1 in, 1 out]
            n292 = property on="SliderSelection" class="Arr (strict)"("Val(Sgnl)"=w330) -> ()  [unwired: 2 in, 2 out]
            n293 = property on="SliderMax" class="Arr (strict)"("Val(Sgnl)"=w329) -> ()  [unwired: 2 in, 2 out]
            n294 = property on="SliderMin" class="Arr (strict)"("Val(Sgnl)"=w328) -> ()  [unwired: 2 in, 2 out]
            n295 = property on="CalPointIDs" class="Arr (strict)"("Val(Sgnl)"=w327) -> ()  [unwired: 2 in, 2 out]
            n296 = Array To Spreadsheet String(delimiter (Tab)=",", array=w331, 3:"%s" ("format string")) -> (spreadsheet string=w334:string)
            n297 = property on="Units" class="Str"("Val(Sgnl)"=w334) -> ()  [unwired: 2 in, 2 out]
            n298 = property on="_Refresh" class="Bool (strict)"("Val(Sgnl)"=TRUE ("Value (Signaling)")) -> ()  [unwired: 2 in, 2 out]
          }
          event "_Data (Hidden)": Value Change {
            n299 = event-data() -> ()  [unwired: 1 in, 6 out]
            n300 = property on="_Refresh" class="Bool (strict)"("Val(Sgnl)"=TRUE ("Value (Signaling)")) -> ()  [unwired: 2 in, 2 out]
          }
        }
      }
    }
  }
